vi "Open Com.vi"(3 "error in (no error)":errorcluster caption="错误输入（无错误）") -> (0 "串口":refnum<visa-resource-name>="COM8", 1 "串口状态":bool, 2 "串口状态":string="串口已连接！")   [LabVIEW 2016]
uses:
  Controls/Global.vi
  <vilib>/Instr/_visa.llb/VISA Configure Serial Port (Instr).vi
panel:
  out "status":bool
  out "VISA resource name out":refnum<visa-resource-name>="COM8"
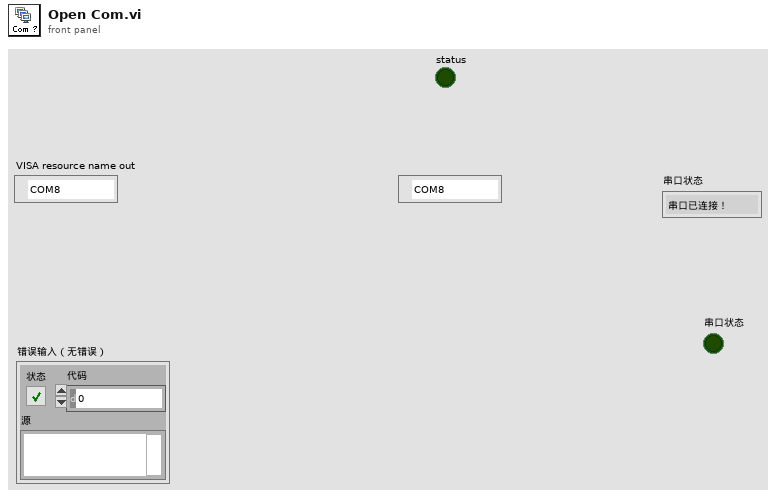
[diagram p1: front panel]
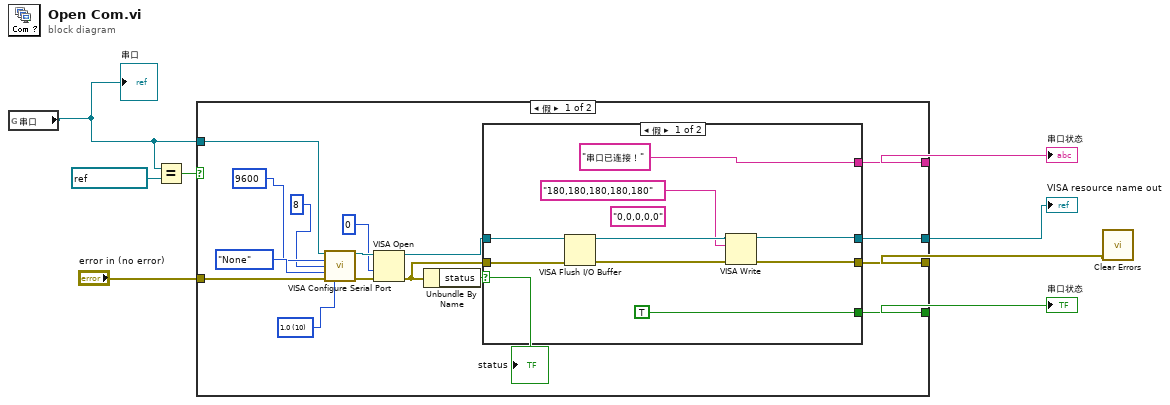
[diagram p0: block diagram]
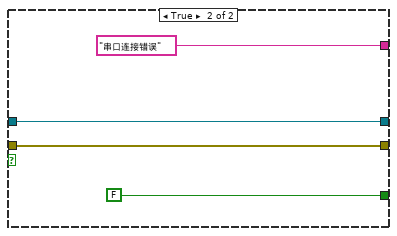
[diagram p2: hidden frame]
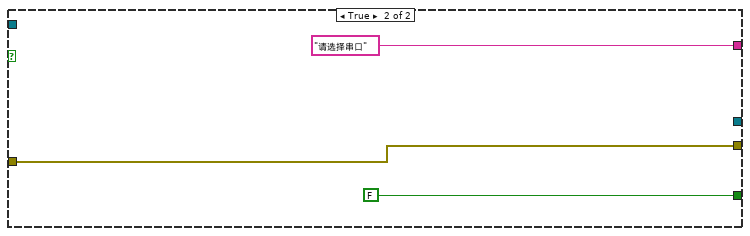
[diagram p3: hidden frame]
diagram:
  n1 = global read "Global.vi" "串口"() -> (w1:refnum<visa-resource-name>)
  "串口" <- w1
  n2 = Equal?(x=w1, y=refnum<visa-resource-name> "无设备！" ("串口")) -> (x = y?=w8:bool)
  n3 = case shown="假" w8 {
    tunnel: [w20 "请选择串口" ("值")] -> w7
    tunnel: [w19 FALSE ("值")] -> w6
    tunnel: [w17 _] -> w5
    tunnel: "error in (no error)" -> [w18 w38]
    tunnel: [w16 w38] -> w2
    tunnel: w1 -> [w12 _]
    frame False {
      w9 = u16 10 items=["1.0"=10, "1.5"=15, "2.0"=20] ("停止位")
      n4 = call-poly "VISA Configure Serial Port"("VISA resource name"=w12, "baud rate (9600)"=u32 9600 ("波特率"), "data bits (8)"=u16 8 ("数据位"), "parity (0:none)"=enum16{"None", "Odd", "Even", "Mark", "Space"}."None", "error in (no error)"=w18, "stop bits (10: 1 bit)"=w9) -> ("VISA resource name out"=w24:refnum<visa-resource-name>, "error out"=w22:errorcluster)  [unwired: 8 in]
      n5 = VISA Open(access mode=u32 0, error in (no error)=w22, VISA resource name=w24) -> (VISA resource name=w15:refnum<visa-resource-name>, error out=w14:errorcluster)  [unwired: 2 in]
      n6 = Unbundle By Name(w14) -> ("status"=w21:bool)
      "status" <- w21
      n7 = case shown="假" w21 {
        tunnel: ["串口已连接！" ("值") "串口连接错误" ("值")] -> w20
        tunnel: [TRUE ("值") FALSE ("值")] -> w19
        tunnel: [w28 w35] -> w17
        tunnel: [w27 w34] -> w16
        tunnel: w15 -> [w31 w35]
        tunnel: w14 -> [w30 w34]
        frame False {
          (unwired) "0,0,0,0,0" ("write buffer")
          n8 = VISA Flush I/O Buffer(VISA resource name=w31, error in (no error)=w30) -> (VISA resource name out=w29:refnum<visa-resource-name>, error out=w26:errorcluster)  [unwired: 1 in]
          n9 = VISA Write(VISA resource name=w29, write buffer="180,180,180,180,180", error in (no error)=w26) -> (VISA resource name out=w28:refnum<visa-resource-name>, error out=w27:errorcluster)  [unwired: 1 out]
        }
        frame True {
        }
      }
    }
    frame True {
    }
  }
  "VISA resource name out" <- w5
  "串口状态" <- w6
  "串口状态" <- w7
  n10 = call <vilib>:"Clear Errors.vi"("error in (no error)"=w2) -> ()  [unwired: 5 in, 2 out]
